vi "KEITHLEY-I-V-Exp.vi"() -> ()   [LabVIEW 2020]
uses:
  <vilib>/Utility/NIReport.llb/Report Type.ctl
  <instrlib>/Keithley 24XX/Public/Data/Read (Single Point).vi
  <vilib>/addons/_office/excel.llb/Excel Easy Table (str).vi
  <instrlib>/Keithley 24XX/Keithley 24XX.lvlib
  <vilib>/Utility/NIReport.llb/NI_ReportGenerationCore.lvlib
  <vilib>/Utility/NIReport.llb/NI_report.lvclass
  <vilib>/addons/_office/NI_ReportGenerationToolkit.lvlib
panel:
  in  "Save Button":bool
  out "error out":errorcluster
  in  "stop 2":bool
  out "XY Graph 3":cluster{"ÇIKIŞ VOLTAJI":dbl[], "AKIM":dbl[]}(graph)
  out "time":dbl[](array[numeric])
  in  "Serial Configuration":T1={"Baud Rate"=9600, "Parity"=0, "Data Bits"=8, "Stop Bits"=10, "Flow Control"=0} {"Flow Control" items=["None", "XON/XOFF", "RTS/CTS", "XON/XOFF & RTS/CTS", "DTR/DSR", "XON/XOFF & DTR/DSR"]; "Stop Bits" items=["1.0"=10, "1.5"=15, "2.0"=20]; "Data Bits" items=["7"=7, "8"=8]; "Parity" items=["None", "Odd", "Even", "Mark", "Space"]; "Baud Rate" items=["300"=300, "600"=600, "1200"=1200, "2400"=2400, "4800"=4800, "9600"=9600, "19200"=19200]}
  in  "VISA resource name":refnum<visa-resource-name>
  out "Table Control":string[][](table)
  out "XY Graph 2":cluster{"ÇIKIŞ VOLTAJI":dbl[], "AKIM":dbl[]}(graph)
  in  "stop":bool
  out "Current":dbl[](array[numeric])
  in  "Step delay time":u32
  in  "Max current value":dbl=0.1
  out "TERİM SAYISI":dbl
  out "Voltage":dbl[](array[numeric])
  in  "Final voltage":dbl
  in  "Increment amount":dbl
  in  "Initial voltage":dbl
  in  "4W AYARI":bool=TRUE
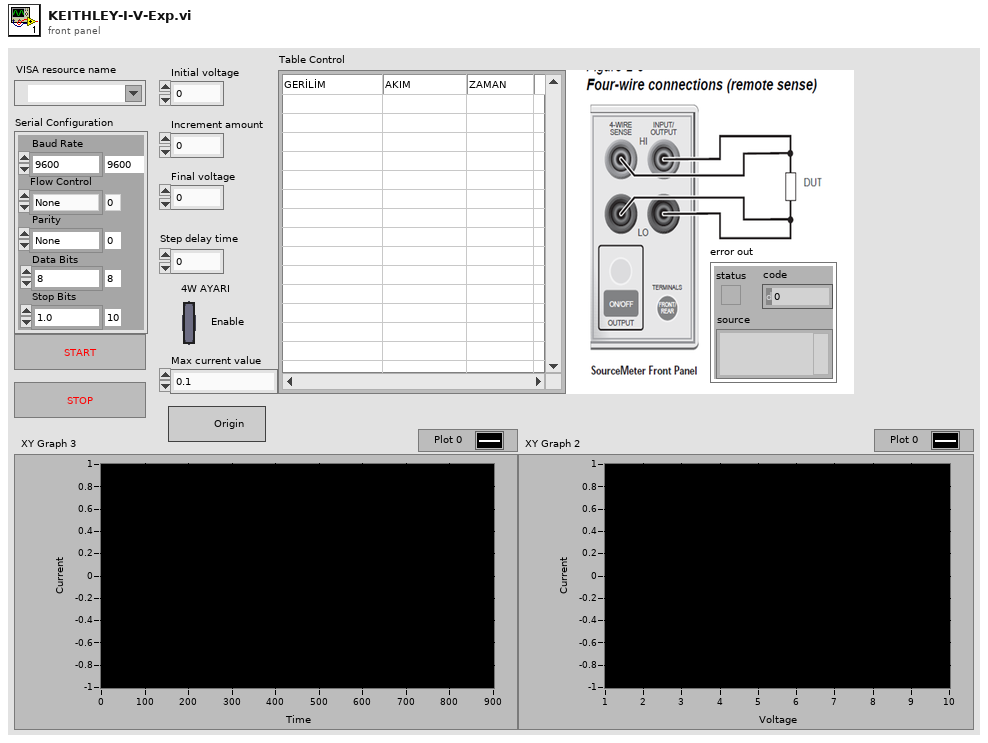
[diagram p1: front panel]
types:
  T1 = cluster{"Baud Rate":u32, "Parity":u16, "Data Bits":u16, "Stop Bits":u16, "Flow Control":u16}
  T2 = typedef "NI_ReportGenerationCore.lvlib/Report Type.ctl" = enum16{"HTML", "Word", "Excel"}
  T3 = enum16{"maximized", "minimized", "normal", "no change"}
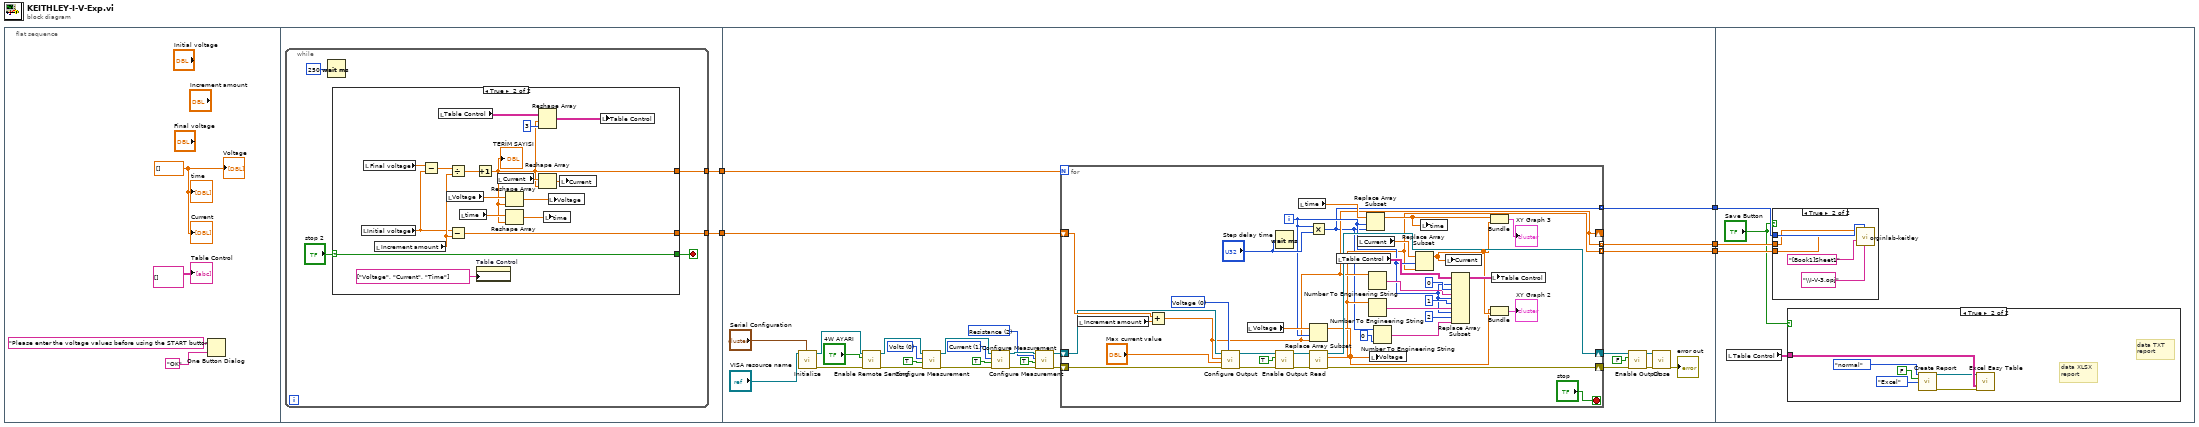
[diagram p0: block diagram]
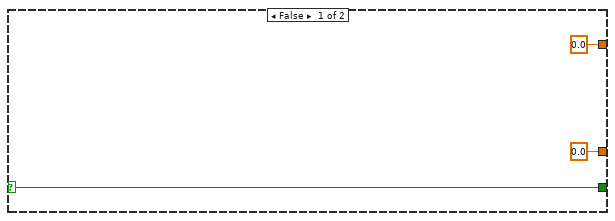
[diagram p2: hidden frame]
diagram:
  n1 = flat-sequence {
    tunnel: [w11] -> w5
    tunnel: [w10] -> w4
    tunnel: w5 -> [w58]
    tunnel: w4 -> [w42]
    tunnel: [w40] -> w3
    tunnel: [w39] -> w2
    tunnel: [w38] -> w1
    tunnel: w3 -> [w108]
    tunnel: w2 -> [w107]
    tunnel: w1 -> [w106]
    frame #0 {
      w9 = dbl[] []
      n2 = One Button Dialog(message="Please enter the voltage values before using the START button.", button name ("OK")="OK") -> ()  [unwired: 1 out]
      "Voltage" <- w9
      "Current" <- w9
      "time" <- w9
      "Table Control" <- string[][] [] ("Table Control")
    }
    frame #1 {
      n3 = while {
        tunnel: [w16] -> w11
        tunnel: [w15] -> w10
        stop <- w13 stop-if-true
        n4 = Wait (ms)(milliseconds to wait=u32 250) -> ()  [unwired: 1 out]
        n5 = case shown="True" "stop 2" {
          selector: "stop 2" -> [w17 w20]
          tunnel: [0.0 w22] -> w16
          tunnel: [0.0 w21] -> w15
          tunnel: [w17 w20] -> w13
          frame False {
          }
          frame True {
            n6 = local read "Initial voltage"() -> (w30:dbl)
            n7 = local read "Final voltage"() -> (w27:dbl)
            n8 = local read "Increment amount"() -> (w31:dbl)
            n9 = Subtract(x=w27, y=w30) -> (x-y=w28:dbl)
            n10 = local read "Table Control"() -> (w34:string[][])
            n11 = local read "Voltage"() -> (w25:dbl[])
            n12 = Divide(x=w28, y=w31) -> (x/y=w29:dbl)
            n13 = Subtract(x=w30, y=w31) -> (x-y=w22:dbl)
            n14 = local read "time"() -> (w36:dbl[])
            n15 = Increment(x=w29) -> (x+1=w21:dbl)
            "TERİM SAYISI" <- w21
            n16 = property on="Table Control" class="Tbl (strict)"("Column Headers[]"=string[] ["Voltage", "Current", "Time"] ("Row Header Strings[]")) -> ()  [unwired: 2 in, 2 out]
            n17 = local read "Current"() -> (w33:dbl[])
            n18 = Reshape Array(w25, w21) -> (w26:dbl[])
            n19 = Reshape Array(w36, w21) -> (w37:dbl[])
            n20 = Reshape Array "Reshape Array"(w34, w21, 3 ("dimension size")) -> (w35:string[][])
            n21 = Reshape Array(w33, w21) -> (w32:dbl[])
            n22 = local write "time"(w37) -> ()
            n23 = local write "Voltage"(w26) -> ()
            n24 = local write "Current"(w32) -> ()
            n25 = local write "Table Control"(w35) -> ()
          }
        }
      }
    }
    frame #2 {
      w48 = u16 2 items=["Volts", "Current", "Resistance"] ("Function (0: Volts)")
      w49 = u16 1 items=["Volts", "Current", "Resistance"] ("Function (0: Volts)")
      w50 = u16 0 items=["Volts", "Current", "Resistance"] ("Function (0: Volts)")
      n26 = call <instrlib>:"Initialize.vi"("Serial Configuration"="Serial Configuration", "VISA resource name"="VISA resource name") -> ("error out"=w66:errorcluster, "VISA resource name out"=w67:refnum<visa-resource-name>)  [unwired: 8 in]
      n27 = call <instrlib>:"Enable Remote Sensing.vi"("error in (no error)"=w66, "Enable Remote Sensing (T: Enable)"="4W AYARI", "VISA resource name"=w67) -> ("error out"=w63:errorcluster, "VISA resource name out"=w64:refnum<visa-resource-name>)  [unwired: 7 in]
      n28 = call <instrlib>:"Configure Measurement.vi"("error in (no error)"=w63, "Enable Auto Range (T:Enable)"=TRUE, "Function (0: Volts)"=w50, "VISA resource name"=w64) -> ("error out"=w61:errorcluster, "VISA resource name out"=w62:refnum<visa-resource-name>)  [unwired: 6 in]
      n29 = call <instrlib>:"Configure Measurement.vi"("error in (no error)"=w61, "Enable Auto Range (T:Enable)"=TRUE, "Function (0: Volts)"=w49, "VISA resource name"=w62) -> ("error out"=w59:errorcluster, "VISA resource name out"=w60:refnum<visa-resource-name>)  [unwired: 6 in]
      n30 = call <instrlib>:"Configure Measurement.vi"("error in (no error)"=w59, "Enable Auto Range (T:Enable)"=TRUE, "Function (0: Volts)"=w48, "VISA resource name"=w60) -> ("error out"=w56:errorcluster, "VISA resource name out"=w57:refnum<visa-resource-name>)  [unwired: 6 in]
      n31 = for {
        N: w42 -> [_]
        shift-right: [w92] -> w51
        shift-left: w57 -> [w98]
        shift-right: [w91] -> w54
        shift-left: w56 -> [w97]
        shift-right: [w70] -> _
        shift-left: w58 -> [w100]
        tunnel: [w70] -> w40 mode=indexing
        tunnel: [w69] -> w39 mode=indexing
        tunnel: [w68] -> w38 mode=indexing
        i -> [w75]
        stop <- "stop" stop-if-true
        w90 = u16 0 items=["Voltage", "Current"] ("Source Mode  (0: Voltage)")
        n32 = local read "Increment amount"() -> (w102:dbl)
        n33 = Add(x=w100, y=w102) -> (x+y=w70:dbl)
        n34 = call <instrlib>:"Configure Output.vi"("Source Mode  (0: Voltage)"=w90, "error in (no error)"=w97, "Compliance  Level (0.1)"="Max current value", "Output Level (0)"=w70, "VISA resource name"=w98) -> ("error out"=w95:errorcluster, "VISA resource name out"=w96:refnum<visa-resource-name>)  [unwired: 5 in]
        n35 = local read "Voltage"() -> (w101:dbl[])
        n36 = Wait (ms)(milliseconds to wait="Step delay time") -> ()  [unwired: 1 out]
        n37 = call <instrlib>:"Enable Output.vi"("error in (no error)"=w95, "Enable Output (T: Enable)"=TRUE, "VISA resource name"=w96) -> ("error out"=w94:errorcluster, "VISA resource name out"=w93:refnum<visa-resource-name>)  [unwired: 7 in]
        n38 = local read "time"() -> (w78:dbl[])
        n39 = Replace Array Subset(array=w101, new element=w70, index=w75) -> (w71:dbl[])
        n40 = call-poly <instrlib>:"Read.vi"("VISA resource name"=w93, "error in (no error)"=w94) -> ("VISA resource name out"=w92:refnum<visa-resource-name>, "Current"=w69:sgl, "error out"=w91:errorcluster)  [unwired: 7 in, 4 out]
        n41 = Multiply(x=w75, y="Step delay time") -> (x*y=w68:u32)
        n42 = local read "Table Control"() -> (w86:string[][])
        n43 = local read "Current"() -> (w89:dbl[])
        n44 = Replace Array Subset(array=w78, new element=w68, index=w75) -> (w77:dbl[])
        n45 = Number To Engineering String(4:w70) -> (0:w82:string)  [unwired: 3 in]
        n46 = Number To Engineering String(4:w69) -> (0:w81:string)  [unwired: 3 in]
        n47 = local write "Voltage"(w71) -> ()
        n48 = Number To Engineering String(2:i16 0 ("precision (6)"), 4:w68) -> (0:w73:string)  [unwired: 2 in]
        n49 = Replace Array Subset(array=w89, new element=w69, index=w75) -> (w79:dbl[])
        n50 = local write "time"(w77) -> ()
        n51 = local write "Current"(w79) -> ()
        n52 = Replace Array Subset(array=w86, new element #1=w82, index (row) #1=w75, index (col) #1=0 ("disabled index (col)"), new element #2=w81, index (row) #2=w75, index (col) #2=1 ("index (col)"), new element #3=w73, index (row) #3=w75, index (col) #3=2 ("disabled index (col)")) -> (w85:string[][])
        n53 = Bundle("time"=w77, "Current"=w79) -> (→"XY Graph 3":cluster{"time":dbl[], "Current":dbl[]})  [unwired: 1 in]
        n54 = Bundle("Voltage"=w71, "Current"=w79) -> (→"XY Graph 2":cluster{"Voltage":dbl[], "Current":dbl[]})  [unwired: 1 in]
        n55 = local write "Table Control"(w85) -> ()
      }
      n56 = call <instrlib>:"Enable Output.vi"("error in (no error)"=w54, "Enable Output (T: Enable)"=FALSE, "VISA resource name"=w51) -> ("error out"=w53:errorcluster, "VISA resource name out"=w52:refnum<visa-resource-name>)  [unwired: 7 in]
      n57 = call <instrlib>:"Close.vi"("error in (no error)"=w53, "VISA resource name"=w52) -> ("error out"=→"error out":errorcluster)  [unwired: 9 in]
    }
    frame #3 {
      n58 = local read "Table Control"() -> (w104:string[][])
      n59 = case shown="True" "Save Button" {
        tunnel: w108 -> [_ w118]
        tunnel: w107 -> [_ w117]
        tunnel: w106 -> [_ w119]
        frame False {
        }
        frame True {
          n60 = call "orginlab-keitley.vi"("\\I-V-2.opj"="\\I-V-3.opj" ("\\I-V-2.opj"), "Zaman"=w119, "[Book1]Sheet1"="[Book1]Sheet1", "Akım"=w117, "Gerilim"=w118) -> ()  [unwired: 7 in]
        }
      }
      n61 = case shown="True" "Save Button" {
        tunnel: w104 -> [_ w111]
        frame False {
        }
        frame True {
          # "data TXT report"
          # "data XLSX report"
          n62 = call <vilib>:"Create Report.vi"("window state (normal)"=T3."normal", "display alerts? (F)"=FALSE, "report type"=Report_Type."Excel") -> ("report out"=w110:refnum<class "NI_report.lvclass">, "error out"=w109:errorcluster)  [unwired: 11 in]
          n63 = call-poly <vilib>:"Excel Easy Table.vi"("report in"=w110, "text data"=w111, "error in (no error)"=w109) -> ()  [unwired: 8 in, 5 out]
        }
      }
    }
  }
